vi "Ratiod.vi"(11 "P":dbl) -> (3 "r":dbl)   [LabVIEW 2020]
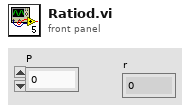
[diagram p1: front panel]
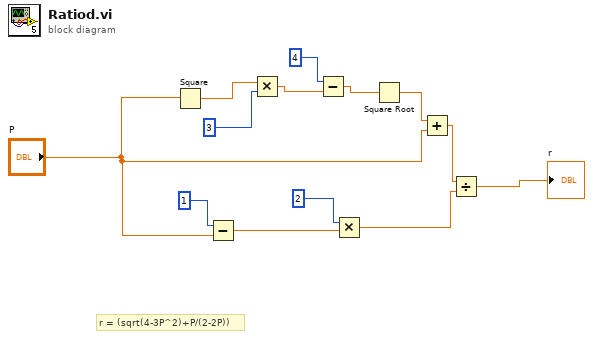
[diagram p0: block diagram]
diagram:
  # "r = (sqrt(4-3P^2)+P/(2-2P))"
  n1 = Square(x="P") -> (x^2=w12:dbl)
  n2 = Subtract(x=1, y="P") -> (x-y=w3:dbl)
  n3 = Multiply(x=w12, y=3) -> (x*y=w10:dbl)
  n4 = Subtract(x=4, y=w10) -> (x-y=w8:dbl)
  n5 = Multiply(x=2, y=w3) -> (x*y=w1:dbl)
  n6 = Square Root(x=w8) -> (sqrt(x)=w7:dbl)
  n7 = Add(x=w7, y="P") -> (x+y=w5:dbl)
  n8 = Divide(x=w5, y=w1) -> (x/y=→"r":dbl)
